vi "Display.vi"() -> ()   [LabVIEW 2017]
panel:
  in  "Scan Mode 2":bool caption="1. Select a Scan Mode:"
  out "Raw":cluster{dbl[], "x+y":dbl[]}(graph)
  out "Calibrated":cluster{dbl[], "x+y":dbl[]}(graph)
  in  "Scan Mode":bool caption="1. Select a Scan Mode:"
  in  "Calibration File:":path=path "G:/t-masIodinedefault.par" caption="2. Choose a Calibration File:"
  out "Calibrated PES":cluster{dbl[], "x+y":dbl[]}(graph)
  out "Calibrated Mass 2":cluster{dbl[], "x+y":dbl[]}(graph)
  in  "FilePath 2":path
  in  "Error In":errorcluster
  out "error out":errorcluster
  # "Mass"
  # "PES"
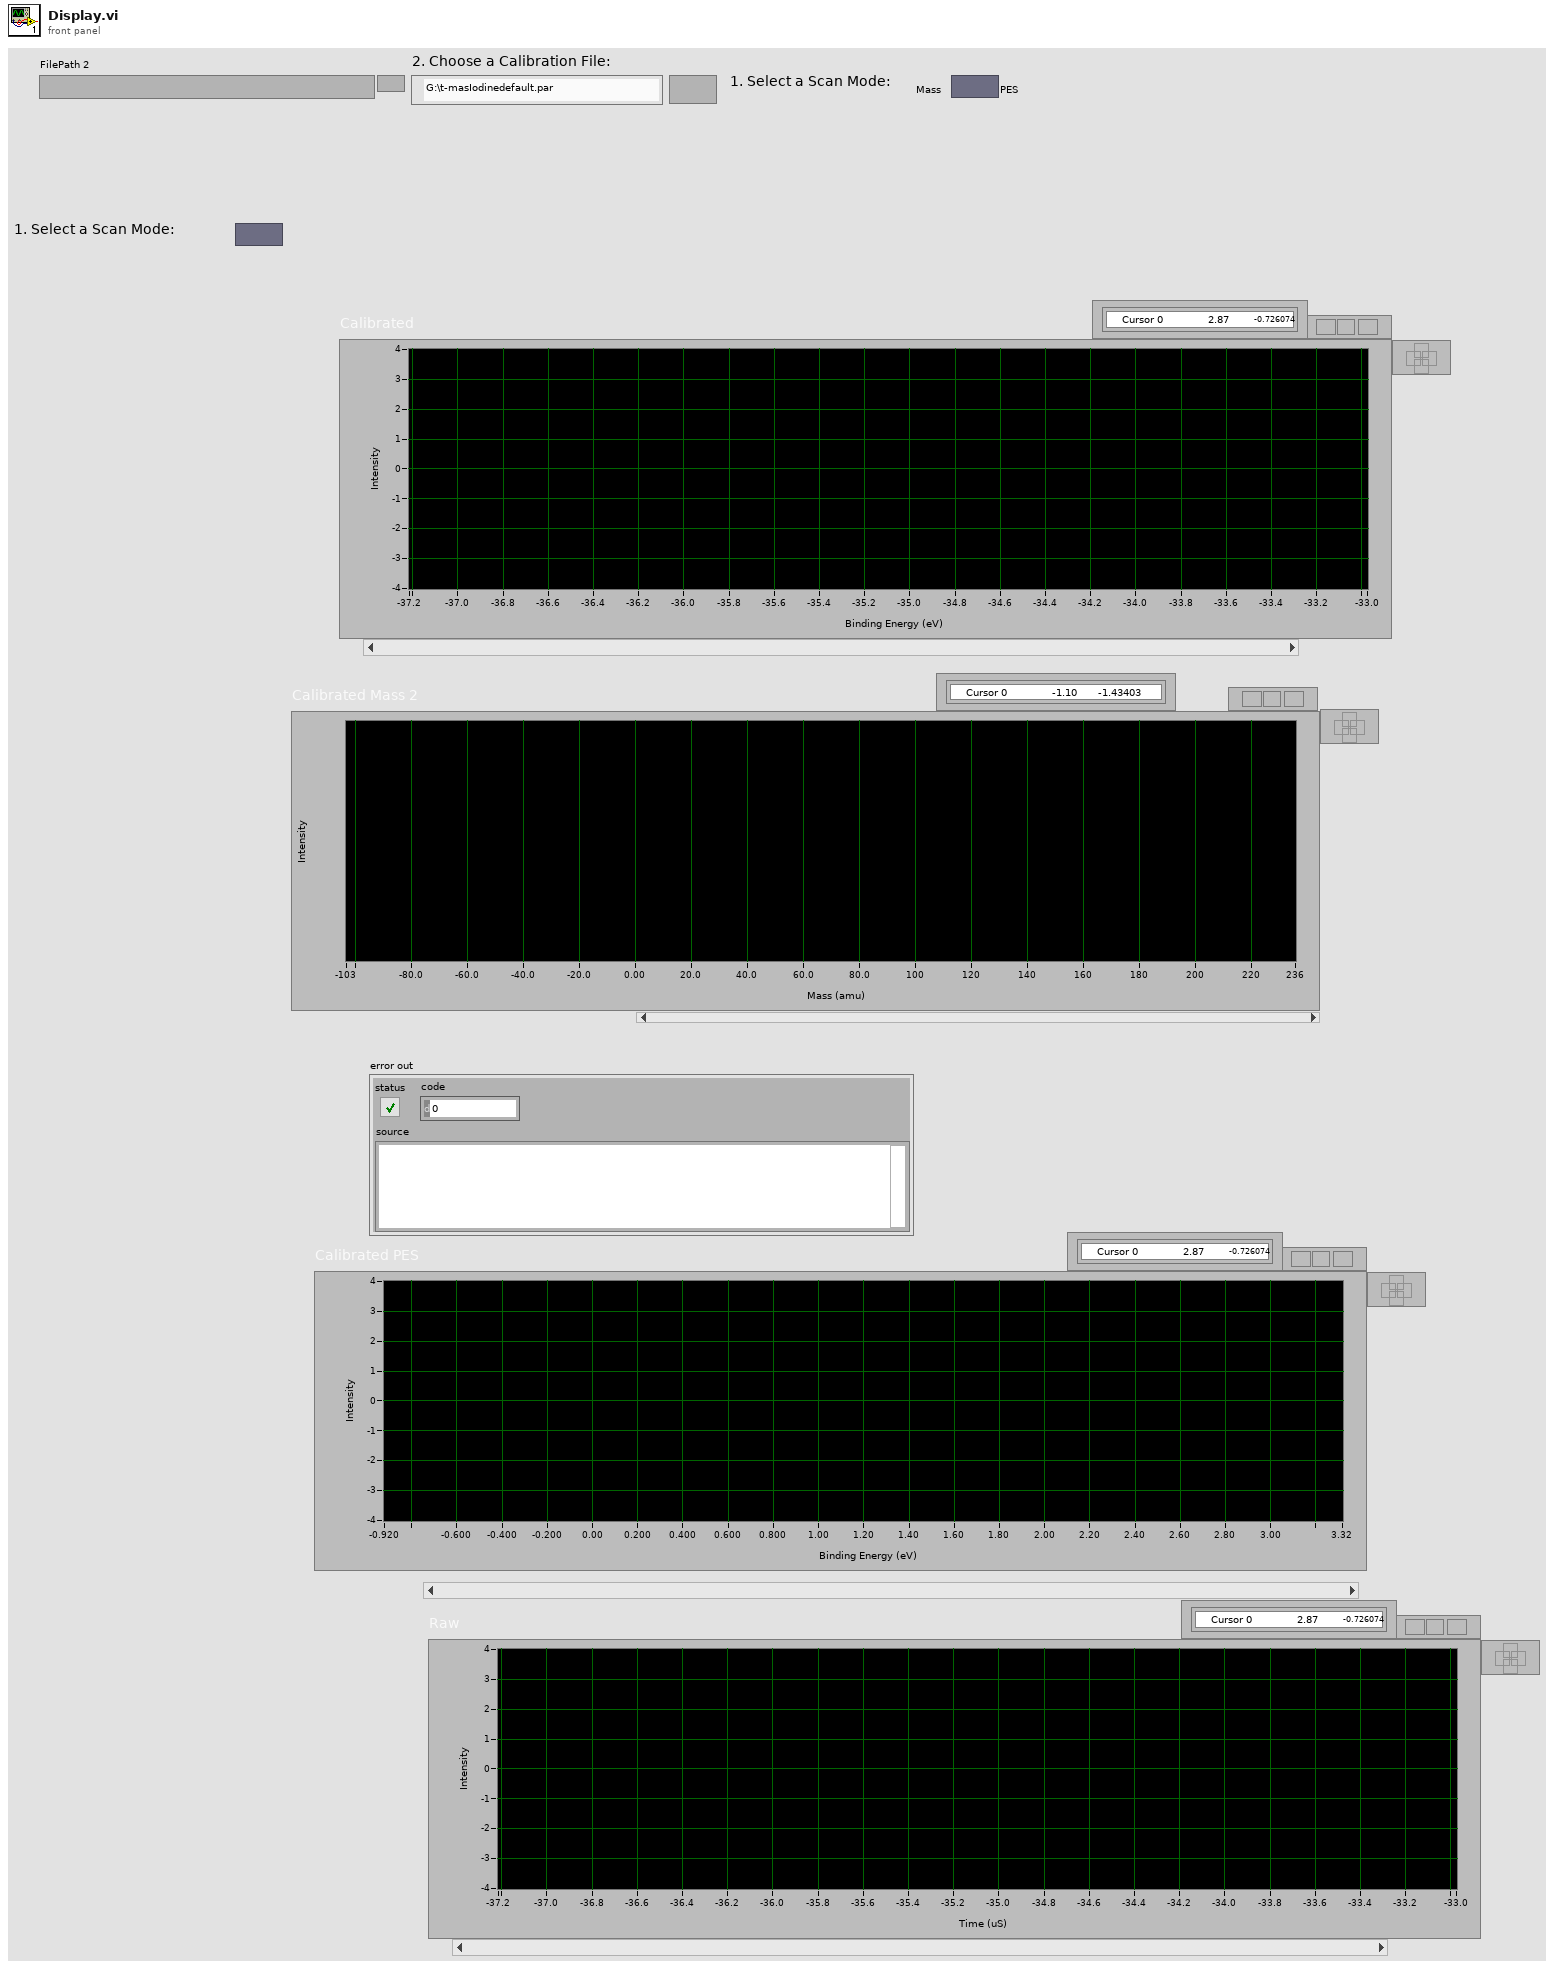
[diagram p1: front panel]
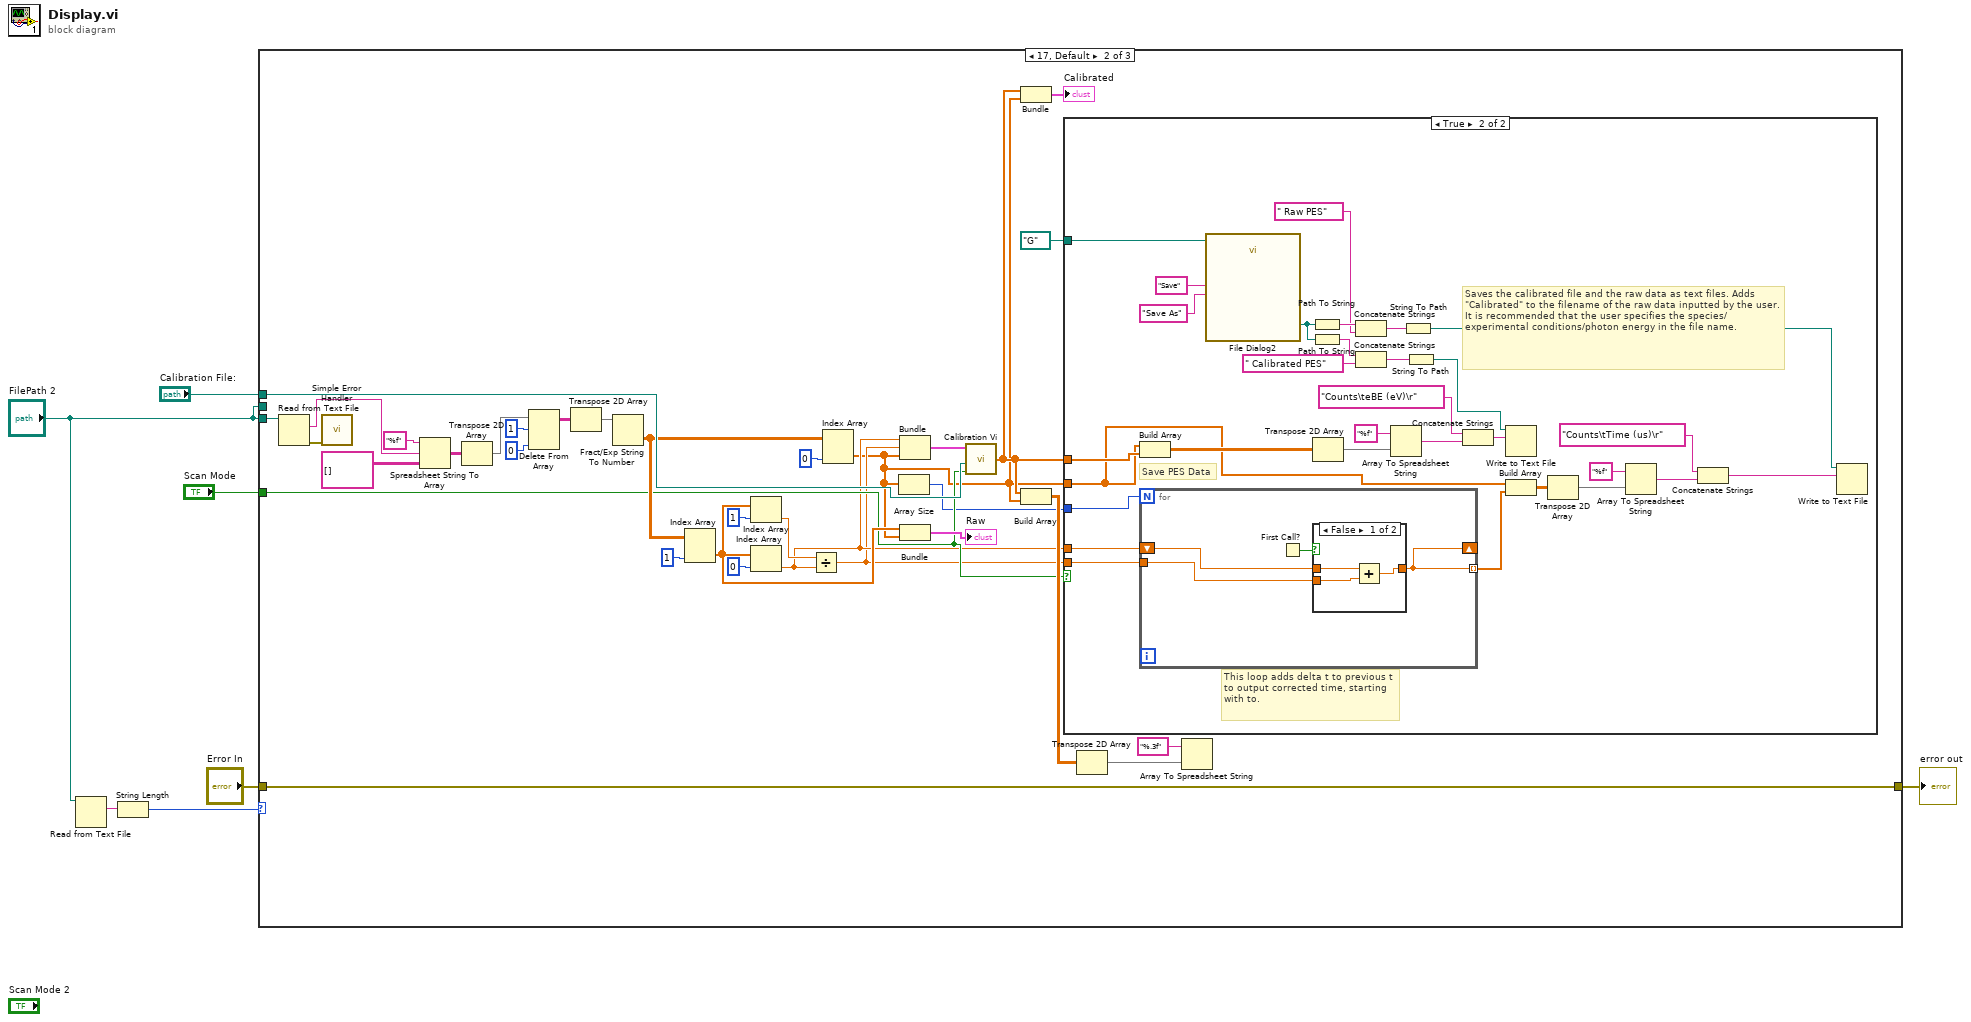
[diagram p0: block diagram]
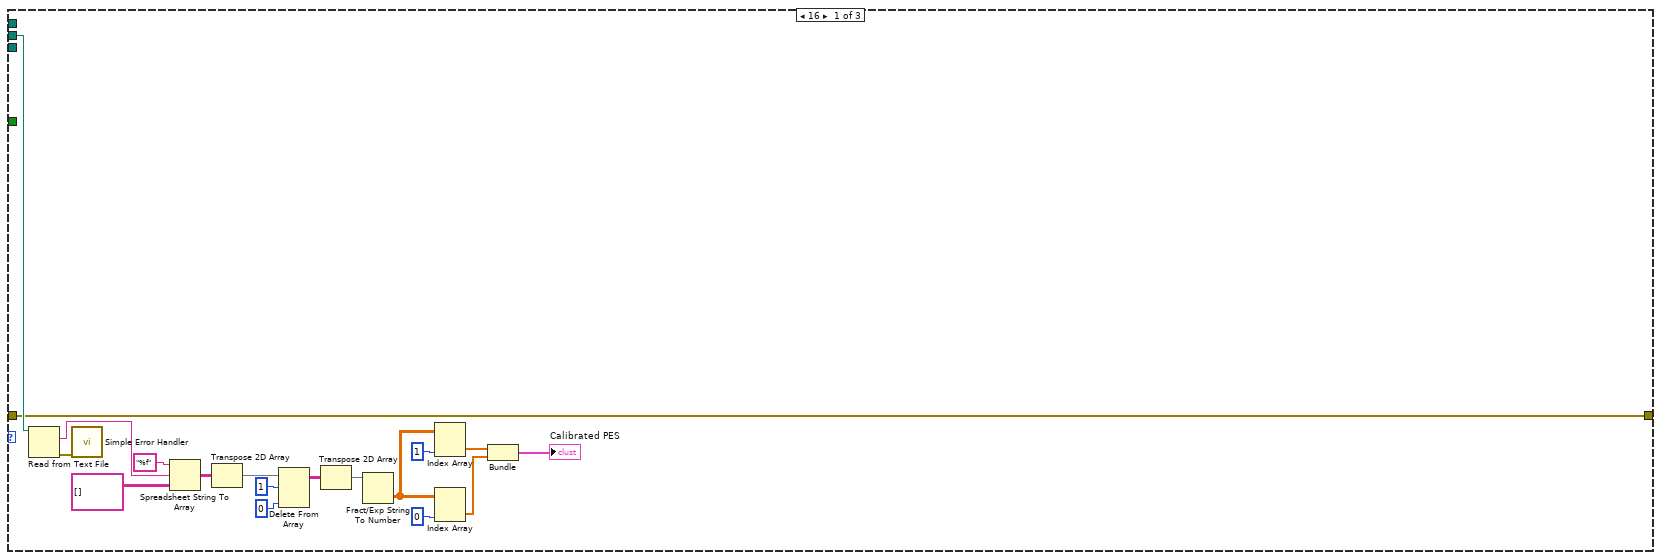
[diagram p2: hidden frame]
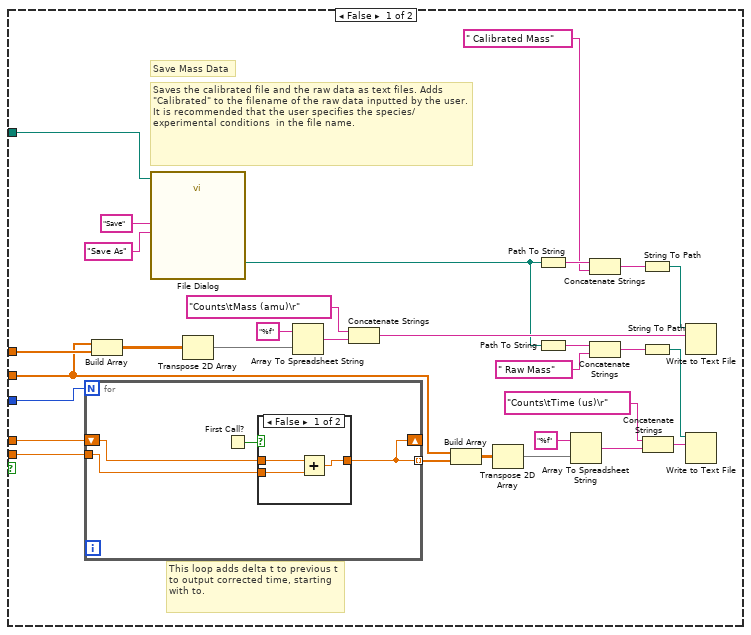
[diagram p3: hidden frame]
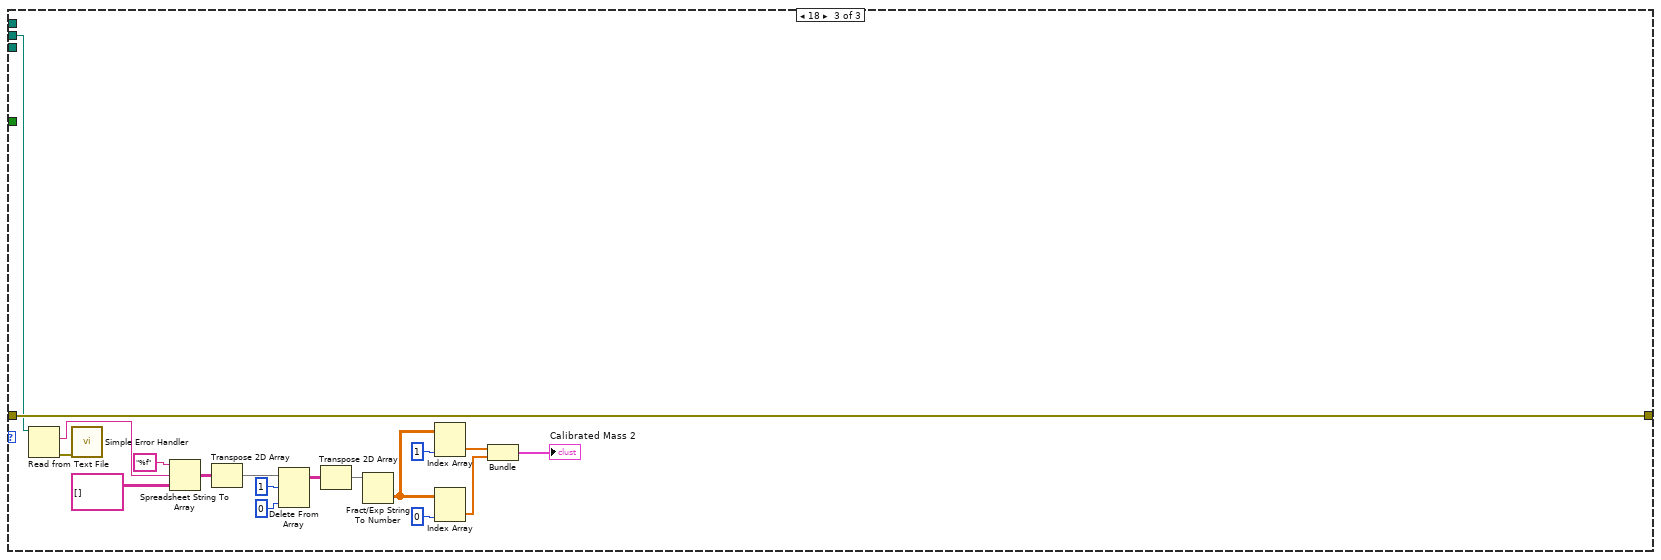
[diagram p6: hidden frame]
diagram:
  n1 = Read from Text File(file (use dialog)="FilePath 2") -> (text=w7:string)  [unwired: 3 in, 3 out]
  n2 = String Length(string=w7) -> (length=w4:i32)
  n3 = case shown="17, Default" w4 {
    tunnel: [w8 w58 w136] -> w5
    tunnel: "Error In" -> [w8 w58 w136]
    tunnel: "FilePath 2" -> [w10 _ w135]
    tunnel: "Scan Mode" -> [_ w32 _]
    tunnel: "Calibration File:" -> [_ w57 _]
    tunnel: "FilePath 2" -> [_ w46 _]
    frame 16 {
      n4 = Read from Text File(file (use dialog)=w10) -> (text=w20:string, error out=w21:errorcluster)  [unwired: 2 in, 3 out]
      n5 = call <vilib>:"Simple Error Handler.vi"("error in (no error)"=w21) -> ()  [unwired: 1 in, 8 out]
      n6 = Spreadsheet String To Array(format string="%f", spreadsheet string=w20, array type (2D Dbl)=string[][] [] ("Array")) -> (array=w19:string[][])  [unwired: 1 in]
      n7 = Transpose 2D Array(2D array=w19) -> (transposed array=w18:string[][])
      n8 = Delete From Array(array=w18, length=1, index (col)=0 ("disabled index (col)")) -> (array with subset deleted=w17:string[][])  [unwired: 1 in, 1 out]
      n9 = Transpose 2D Array(2D array=w17) -> (transposed array=w16:string[][])
      n10 = Fract/Exp String To Number(string=w16) -> (number=w15:dbl[][])  [unwired: 1 in, 3 out]
      n11 = Index Array(array=w15, index (col)=1 ("disabled index (col)")) -> (element=w11:dbl[])  [unwired: 1 in]
      n12 = Index Array(array=w15, index (col)=0 ("disabled index (col)")) -> (element=w12:dbl[])  [unwired: 1 in]
      n13 = Bundle(w11, w12) -> (→"Calibrated PES":cluster{dbl[], dbl[]})  [unwired: 1 in]
    }
    frame 17, Default {
      n14 = Read from Text File(file (use dialog)=w46) -> (text=w51:string, error out=w52:errorcluster)  [unwired: 2 in, 3 out]
      n15 = call <vilib>:"Simple Error Handler.vi"("error in (no error)"=w52) -> ()  [unwired: 1 in, 8 out]
      n16 = Spreadsheet String To Array(format string="%f", spreadsheet string=w51, array type (2D Dbl)=string[][] [] ("Array")) -> (array=w50:string[][])  [unwired: 1 in]
      n17 = Transpose 2D Array(2D array=w50) -> (transposed array=w49:string[][])
      n18 = Delete From Array(array=w49, length=1, index (col)=0 ("disabled index (col)")) -> (array with subset deleted=w48:string[][])  [unwired: 1 in, 1 out]
      n19 = Transpose 2D Array(2D array=w48) -> (transposed array=w47:string[][])
      n20 = Fract/Exp String To Number(string=w47) -> (number=w44:dbl[][])  [unwired: 1 in, 3 out]
      n21 = Index Array(array=w44, index (col)=1 ("disabled index (col)")) -> (element=w34:dbl[])  [unwired: 1 in]
      n22 = Index Array(array=w34, index=1) -> (element=w40:dbl)
      n23 = Index Array(array=w34, index=0) -> (element=w29:dbl)
      n24 = Divide(x=w40, y=w29) -> (x/y=w28:dbl)
      n25 = Index Array(array=w44, index (col)=0 ("disabled index (col)")) -> (element=w26:dbl[])  [unwired: 1 in]
      n26 = Array Size(array=w26) -> (size(s)=w27:i32)
      n27 = Bundle("String"=w29, w28, w26) -> (w39:cluster{"String":dbl, dbl, dbl[]})  [unwired: 1 in]
      n28 = Bundle(w34, w26) -> (→"Raw":cluster{dbl[], dbl[]})  [unwired: 1 in]
      n29 = call "Calibration Vi.vi"("Scan Mode"=w32, "start path"=w57, "Summation Graph"=w39) -> ("Calibrated x-data"=w30:dbl[])  [unwired: 1 in]
      n30 = Bundle("Calibrated x-data"=w30, w26) -> (→"Calibrated":cluster{"Calibrated x-data":dbl[], dbl[]})  [unwired: 1 in]
      n31 = Build Array(w30, w26) -> (w36:dbl[][])
      n32 = case shown="True" w32 {
        tunnel: path "G:/" ("start path") -> [w67 w110]
        tunnel: w30 -> [w65 w104]
        tunnel: w26 -> [w61 w97]
        tunnel: w29 -> [w60 w100]
        tunnel: w28 -> [w59 w99]
        tunnel: w27 -> [w62 w98]
        frame False {
          # "Save Mass Data"
          # "This loop adds delta t to previous t to output corrected time, starting with to."
          # "Saves the calibrated file and the raw data as text files. Adds \"Calibrated\" to the filename of the raw data inputted by the user. It is recommended that the user specifies the species/experimental conditions  in the file name."
          n33 = for {
            N: w62 -> [_]
            tunnel: w59 -> [w91]
            shift-right: [w89] -> _
            shift-left: w60 -> [w92]
            tunnel: [w89] -> w68 mode=indexing
            n34 = First Call?() -> (First Call?: T/F=w90:bool)
            n35 = case shown="False" w90 {
              tunnel: w92 -> [w94 w96]
              tunnel: [w95 w96] -> w89
              tunnel: w91 -> [w93 _]
              frame False {
                n36 = Add(x=w94, y=w93) -> (x+y=w95:dbl)
              }
              frame True {
              }
            }
          }
          n37 = Build Array(w61, w65) -> (w76:dbl[][])
          n38 = call "File Dialog"("start path"=w67, "prompt"="Save As", "button label"="Save") -> ("selected path"=w63:path)  [unwired: 9 in, 3 out]
          n39 = Transpose 2D Array(2D array=w76) -> (transposed array=w66:dbl[][])
          n40 = Array To Spreadsheet String(array=w66, 3:"%f" ("format string")) -> (spreadsheet string=w74:string)  [unwired: 1 in]
          n41 = Concatenate Strings("Counts\tMass (amu)\r", w74) -> (w73:string)
          n42 = Build Array(w61, w68) -> (w88:dbl[][])
          n43 = Transpose 2D Array(2D array=w88) -> (transposed array=w87:dbl[][])
          n44 = Path To String(path=w63) -> (string=w80:string)
          n45 = Path To String(path=w63) -> (string=w71:string)
          n46 = Array To Spreadsheet String(array=w87, 3:"%f" ("format string")) -> (spreadsheet string=w84:string)  [unwired: 1 in]
          n47 = Concatenate Strings(w80, " Calibrated Mass" ("string")) -> (w78:string)
          n48 = Concatenate Strings(w71, " Raw Mass" ("string")) -> (w69:string)
          n49 = String To Path(string=w78) -> (path=w77:path)
          n50 = String To Path(string=w69) -> (path=w64:path)
          n51 = Concatenate Strings("Counts\tTime (us)\r", w84) -> (w83:string)
          n52 = Write to Text File(file (use dialog)=w77, text=w73) -> ()  [unwired: 2 in, 3 out]
          n53 = Write to Text File(file (use dialog)=w64, text=w83) -> ()  [unwired: 2 in, 3 out]
        }
        frame True {
          # "Save PES Data"
          # "This loop adds delta t to previous t to output corrected time, starting with to."
          # "Saves the calibrated file and the raw data as text files. Adds \"Calibrated\" to the filename of the raw data inputted by the user. It is recommended that the user specifies the species/experimental conditions/photon energy in the file name."
          n54 = Build Array(w97, w104) -> (w115:dbl[][])
          n55 = for {
            N: w98 -> [_]
            tunnel: w99 -> [w129]
            shift-right: [w127] -> _
            shift-left: w100 -> [w130]
            tunnel: [w127] -> w103 mode=indexing
            n56 = First Call?() -> (First Call?: T/F=w128:bool)
            n57 = case shown="False" w128 {
              tunnel: w130 -> [w132 w134]
              tunnel: [w133 w134] -> w127
              tunnel: w129 -> [w131 _]
              frame False {
                n58 = Add(x=w132, y=w131) -> (x+y=w133:dbl)
              }
              frame True {
              }
            }
          }
          n59 = call "File Dialog2"("start path"=w110, "prompt"="Save As", "button label"="Save") -> ("selected path"=w105:path)  [unwired: 9 in, 3 out]
          n60 = Path To String(path=w105) -> (string=w108:string)
          n61 = Path To String(path=w105) -> (string=w119:string)
          n62 = Transpose 2D Array(2D array=w115) -> (transposed array=w114:dbl[][])
          n63 = Concatenate Strings(w108, " Raw PES" ("string")) -> (w106:string)
          n64 = Concatenate Strings(w119, " Calibrated PES" ("string")) -> (w117:string)
          n65 = Array To Spreadsheet String(array=w114, 3:"%f" ("format string")) -> (spreadsheet string=w112:string)  [unwired: 1 in]
          n66 = String To Path(string=w106) -> (path=w101:path)
          n67 = String To Path(string=w117) -> (path=w116:path)
          n68 = Concatenate Strings("Counts\teBE (eV)\r", w112) -> (w111:string)
          n69 = Write to Text File(file (use dialog)=w116, text=w111) -> ()  [unwired: 2 in, 3 out]
          n70 = Build Array(w97, w103) -> (w126:dbl[][])
          n71 = Transpose 2D Array(2D array=w126) -> (transposed array=w125:dbl[][])
          n72 = Array To Spreadsheet String(array=w125, 3:"%f" ("format string")) -> (spreadsheet string=w122:string)  [unwired: 1 in]
          n73 = Concatenate Strings("Counts\tTime (us)\r", w122) -> (w121:string)
          n74 = Write to Text File(file (use dialog)=w101, text=w121) -> ()  [unwired: 2 in, 3 out]
        }
      }
      n75 = Transpose 2D Array(2D array=w36) -> (transposed array=w35:dbl[][])
      n76 = Array To Spreadsheet String(array=w35, 3:"%.3f") -> ()  [unwired: 2 out]
    }
    frame 18 {
      n77 = Read from Text File(file (use dialog)=w135) -> (text=w147:string, error out=w148:errorcluster)  [unwired: 2 in, 3 out]
      n78 = call <vilib>:"Simple Error Handler.vi"("error in (no error)"=w148) -> ()  [unwired: 1 in, 8 out]
      n79 = Spreadsheet String To Array(format string="%f", spreadsheet string=w147, array type (2D Dbl)=string[][] [] ("Array")) -> (array=w146:string[][])  [unwired: 1 in]
      n80 = Transpose 2D Array(2D array=w146) -> (transposed array=w145:string[][])
      n81 = Delete From Array(array=w145, length=1, index (col)=0 ("disabled index (col)")) -> (array with subset deleted=w144:string[][])  [unwired: 1 in, 1 out]
      n82 = Transpose 2D Array(2D array=w144) -> (transposed array=w143:string[][])
      n83 = Fract/Exp String To Number(string=w143) -> (number=w142:dbl[][])  [unwired: 1 in, 3 out]
      n84 = Index Array(array=w142, index (col)=1 ("disabled index (col)")) -> (element=w138:dbl[])  [unwired: 1 in]
      n85 = Index Array(array=w142, index (col)=0 ("disabled index (col)")) -> (element=w139:dbl[])  [unwired: 1 in]
      n86 = Bundle(w138, w139) -> (→"Calibrated Mass 2":cluster{dbl[], dbl[]})  [unwired: 1 in]
    }
  }
  "error out" <- w5
